vi "robotFollowsHuman.vi"() -> ()   [LabVIEW 2012]
doc: "Simple demonstration of the Kinesthesia toolkit which allows user to conect the Kinect sensor to LabVIEW"
uses:
  <vilib>/LabVIEW Interface for Arduino/Type Defs/Connection Type.ctl
  E:/Kinect/Neobotix/CSInterface/RosBridgeDotNet.dll
  RosBridgeDotNet.dll
  <vilib>/University of Leeds/Kinesthesia Toolkit for Microsoft Kinect/_Polymorphic Close/Close-Skeleton and Video.vi
  <vilib>/University of Leeds/Kinesthesia Toolkit for Microsoft Kinect/_Polymorphic Configure/Event-Skeleton and Video.vi
  <vilib>/University of Leeds/Kinesthesia Toolkit for Microsoft Kinect/_Polymorphic Read/Read-Skeleton and Video.vi
  <vilib>/LabVIEW Interface for Arduino/LabVIEW Interface for Arduino.lvlib
panel:
  in  "Sebesseg":dbl(slide)=1.5254237288135593 scale=1.0..3.0
  in  "Mozog":bool=TRUE
  out "error out":errorcluster
  in  "r":bool
  in  "g":bool
  in  "b":bool
  out "Táv":dbl(slide) scale=0.0..1.4
  out "Szög":dbl(knob)
  out "XY Graph":cluster{"X":dbl[], "Y":dbl[]}[](graph)
  out "y":dbl
  out "x":dbl
  out "Connected":bool
  out "pingelhet":bool
  out "Error Out":errorcluster
  out "Jobb":dbl(slide) scale=-4.0..4.0
  out "Bal":dbl(slide) scale=-4.0..4.0 scale format="%0#1_1g"
  out "2D Picture":picture
  out "3D Skeleton":refnum<vi>(3d-picture)
  in  "stop":bool
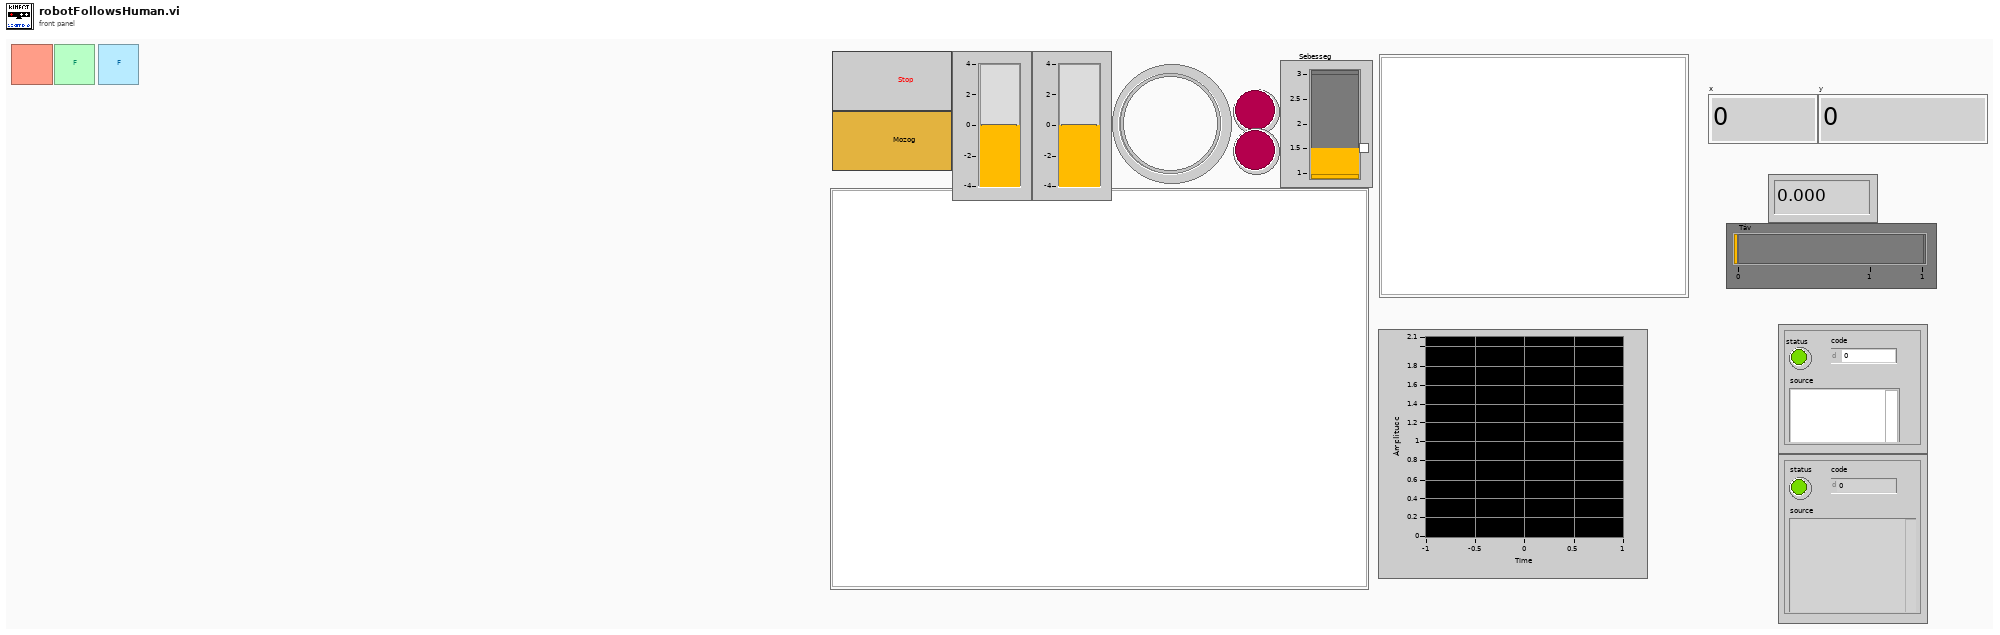
[diagram p1: front panel]
types:
  T1 = typedef "LabVIEW Interface for Arduino.lvlib/Connection Type.ctl" = enum8{"USB / Serial", "XBEE", "BlueSmirf (Bluetooth)"}
  T2 = cluster{cluster{"reference out":refnum<k24>, "KinectSensors":refnum<k24>}, "get_Item":refnum<k24>}
  T3 = cluster{"reference out":refnum<k24>, "KinectSensors":refnum<k24>, "SkeletonStream":refnum<k24>, "ColorStream":refnum<k24>, refnum<k24>[], "get_Item":refnum<k24>}
  T4 = cluster{"Scene":refnum<vi>, "Joints":refnum<vi>[], "Bones":refnum<vi>[]}
  T5 = typedef "LabVIEW Interface for Arduino.lvlib/Arduino Resource.ctl" = cluster{"VISA resource":refnum<visa-resource-name>, "Board Type":T6, "Connection Type":enum8{"USB / Serial"}, "Bytes Per Packet (15)":u8}
  T6 = typedef "LabVIEW Interface for Arduino.lvlib/Board Type.ctl" = enum16{"Uno", "Dimuelanove w/Atmega 328", "Mega 2560"}
  T7 = enum16{"hip centre", "spine", "shoulder centre", "head", "shoulder left", "elbow left", "wrist left", "hand left", "shoulder right", "elbow right", "wrist right", "hand right", "hip left", "knee left", "ankle left", "foot left", "hip right", "knee right", "ankle right", "foot right"}
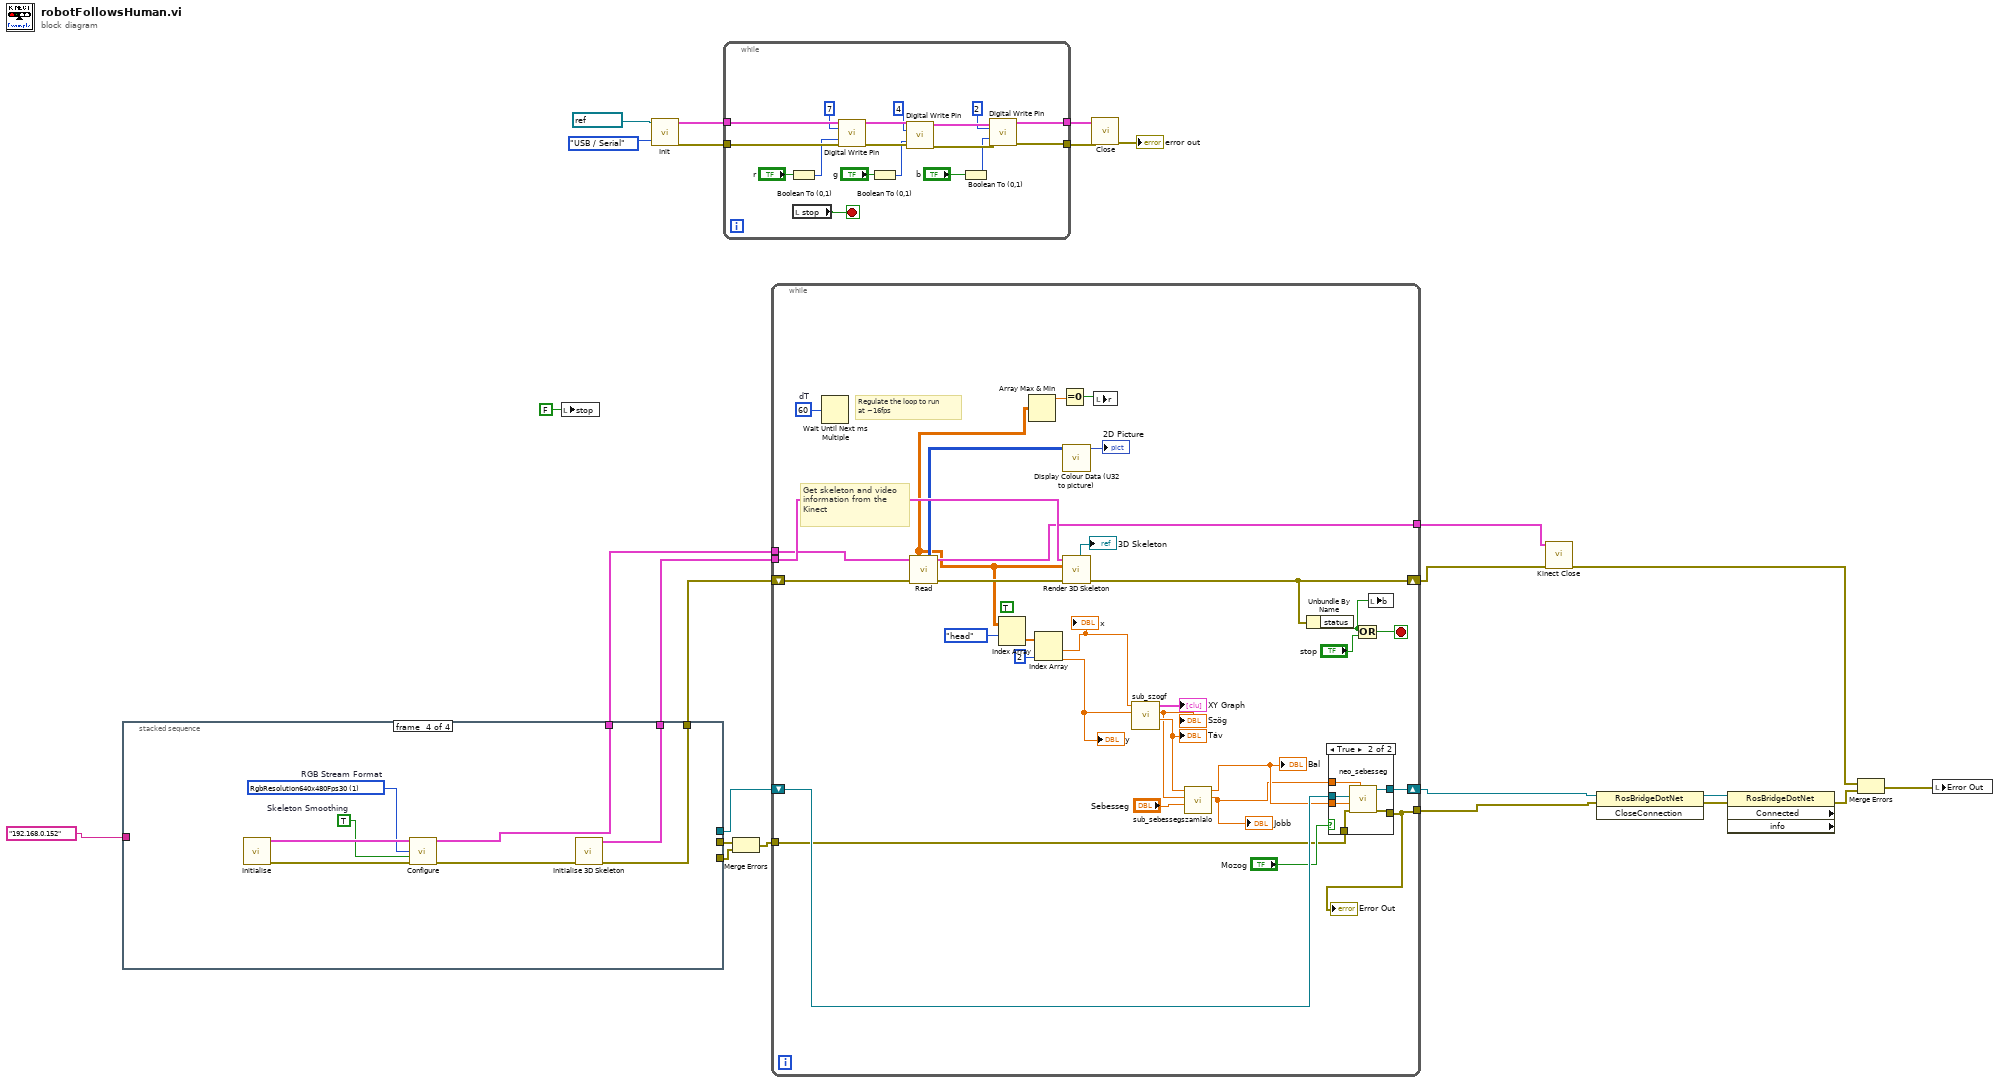
[diagram p0: block diagram]
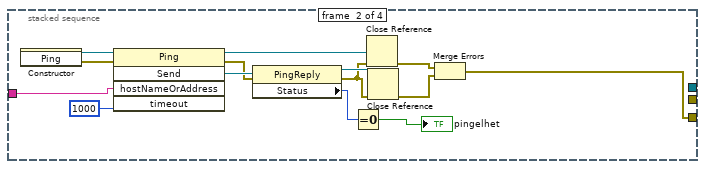
[diagram p3: hidden frame]
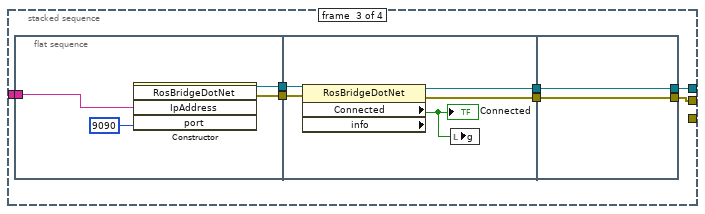
[diagram p4: hidden frame]
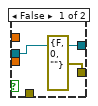
[diagram p5: hidden frame]
diagram:
  n1 = stacked-sequence {
    tunnel: "192.168.0.152" ("IpAddress") -> [_ w33 w42 _]
    tunnel: [_ _ w41 _] -> w21
    tunnel: [_ _ w40 _] -> w9
    tunnel: [_ w26 _ _] -> w7
    tunnel: [_ _ _ w60] -> w6
    tunnel: [_ _ _ w59] -> w5
    tunnel: [_ _ _ w58] -> w4
    frame #0 {
    }
    frame #1 {
      n2 = constructor class="Ping"() -> (reference out=w38:refnum<k24>, error out=w30:errorcluster)  [unwired: 3 in, 1 out]
      n3 = invoke class="Ping" method="Send"(reference=w38, error in=w30, "hostNameOrAddress"=w33, "timeout"=1000) -> (reference out=w36:refnum<k24>, error out=w31:errorcluster, "Send"=w39:refnum<k24>)  [unwired: 1 in, 2 out]
      n4 = property class="PingReply"(reference=w39, error in=w31) -> (reference out=w37:refnum<k24>, error out=w29:errorcluster, "Status"=w34:i32)
      n5 = Equal To 0?(x=w34) -> (x = 0?=→"pingelhet":bool)
      n6 = Close Reference(reference=w36, error in (no error)=w29) -> (error out=w28:errorcluster)
      n7 = Close Reference(reference=w37, error in (no error)=w29) -> (error out=w27:errorcluster)
      n8 = Merge Errors(w28, w27) -> (w26:errorcluster)
    }
    frame #2 {
      n9 = flat-sequence {
        tunnel: [w49] -> w46
        tunnel: [w48] -> w45
        tunnel: w42 -> [w47]
        tunnel: w46 -> [w55]
        tunnel: w45 -> [w54]
        tunnel: [w53] -> w44
        tunnel: [w52] -> w43
        tunnel: w44 -> [w56]
        tunnel: w43 -> [w57]
        tunnel: [w57] -> w40
        tunnel: [w56] -> w41
        frame #0 {
          n10 = constructor class="RosBridgeDotNet"("IpAddress"=w47, "port"=9090) -> (reference out=w49:refnum<k24>, error out=w48:errorcluster)  [unwired: 3 in, 3 out]
        }
        frame #1 {
          n11 = property class="RosBridgeDotNet" props=["Connected", "info"](reference=w55, error in=w54) -> (reference out=w53:refnum<k24>, error out=w52:errorcluster, "Connected"=w51:bool)  [unwired: 1 out]
          "Connected" <- w51
          n12 = local write "g"(w51) -> ()
        }
        frame #2 {
        }
      }
    }
    frame #3 {
      w62 = 1 items=["Undefined", "RgbResolution640x480Fps30", "RgbResolution1280x960Fps12", "YuvResolution640x480Fps15", "RawYuvResolution640x480Fps15"]  # RGB Stream Format
      w63 = TRUE  # Skeleton Smoothing
      n13 = call <vilib>:"Initialise.vi"() -> ("Kinect References out"=w65:T2, "error out"=w64:errorcluster)  [unwired: 14 in]
      n14 = call-poly <vilib>:"Configure.vi"("Kinect References in"=w65, "RGB Stream Format"=w62, "Skeleton Smoothing"=w63, "error in"=w64) -> ("Kinect References out"=w59:T3, "error out"=w61:errorcluster)  [unwired: 10 in]
      n15 = call <vilib>:"Initialise 3D Skeleton.vi"("error in (no error)"=w61) -> ("error out"=w58:errorcluster, "Scene & Skeleton Refs"=w60:T4)  [unwired: 9 in]
    }
  }
  n16 = local write "stop"(FALSE ("stop")) -> ()
  n17 = call <vilib>:"Init.vi"("VISA resource"=refnum<visa-resource-name> "COM3" ("visares"), "Connection Type (USB/Serial)"=Connection_Type."USB / Serial") -> ("Arduino Resource"=w14:T5, "error out"=w13:errorcluster)  [unwired: 16 in]
  n18 = while {
    tunnel: w14 -> [w83]
    tunnel: [w75] -> w11
    tunnel: w13 -> [w82]
    tunnel: [w76] -> w10
    stop <- w66 stop-if-true
    n19 = Boolean To (0,1)(Boolean="r") -> (0, 1=w71:i16)
    n20 = local read "stop"() -> (w66:bool)
    n21 = call <vilib>:"Digital Write Pin.vi"("Arduino Resource"=w83, "Digital I/O Pin (0)"=u8 7, "Value (0)"=w71, "error in"=w82) -> ("Arduino Resource"=w80:T5, "error out"=w79:errorcluster)  [unwired: 10 in]
    n22 = Boolean To (0,1)(Boolean="g") -> (0, 1=w68:i16)
    n23 = call <vilib>:"Digital Write Pin.vi"("Arduino Resource"=w80, "Digital I/O Pin (0)"=u8 4, "Value (0)"=w68, "error in"=w79) -> ("Arduino Resource"=w78:T5, "error out"=w77:errorcluster)  [unwired: 10 in]
    n24 = Boolean To (0,1)(Boolean="b") -> (0, 1=w67:i16)
    n25 = call <vilib>:"Digital Write Pin.vi"("Arduino Resource"=w78, "Digital I/O Pin (0)"=u8 2, "Value (0)"=w67, "error in"=w77) -> ("Arduino Resource"=w75:T5, "error out"=w76:errorcluster)  [unwired: 10 in]
  }
  n26 = Merge Errors(w9, w7) -> (w8:errorcluster)
  n27 = while {
    tunnel: [w106] -> w24
    tunnel: w6 -> [w115]
    tunnel: w5 -> [w107]
    shift-right: [w108] -> w25
    shift-left: w4 -> [w105]
    shift-right: [w100] -> w20
    shift-left: w21 -> [w101]
    tunnel: [w99] -> w19
    tunnel: w8 -> [w85]
    stop <- w109 stop-if-true
    (unwired) TRUE ("Custom Coordinates Instead of Joint 2")
    w113 = u32 60  # dT
    # "Get skeleton and video\ninformation from the Kinect"
    # "Regulate the loop to run\nat ~16fps"
    n28 = Wait Until Next ms Multiple(millisecond multiple=w113) -> ()  [unwired: 1 out]
    n29 = call-poly <vilib>:"Read.vi"("Kinect References in"=w107, "error in (no error)"=w105) -> ("Primary Skeleton Array"=w92:dbl[][], "Colour output array (U24, RGB)"=w93:u32[][], "Kinect References out"=w106:T3, "error out"=w111:errorcluster)  [unwired: 9 in, 1 out]
    n30 = Index Array(array=w92, index (row)=T7."head" ("Joint 1")) -> (element=w103:dbl[])  [unwired: 1 in]
    n31 = Array Max & Min(array=w92) -> (max value=w91:dbl)  [unwired: 3 out]
    n32 = Index Array(array=w103, index #2=2 ("index")) -> (element #1=w98:dbl, element #2=w97:dbl)  [unwired: 1 in]
    "x" <- w98
    "y" <- w97
    n33 = Equal To 0?(x=w91) -> (x = 0?=w90:bool)
    n34 = call <vilib>:"Display Colour Data (U32 to picture).vi"("Colour output array (U24, RGB)"=w93) -> ("new picture"=→"2D Picture":picture)  [unwired: 10 in]
    n35 = call <vilib>:"Render 3D Skeleton.vi"("error in (no error)"=w111, "Array of Joint Positions"=w92, "Scene & Skeleton Refs In"=w115) -> ("error out"=w108:errorcluster, "Scene Out"=→"3D Skeleton":refnum<vi>)  [unwired: 5 in, 2 out]
    n36 = local write "r"(w90) -> ()
    n37 = call "sub_szogf.vi"("y"=w97, "x"=w98) -> ("Táv"=w95:dbl, "SzögNulllpont"=w94:dbl, "XY Graph"=→"XY Graph":cluster{"X":dbl[], "Y":dbl[]}[])  [unwired: 7 in]
    "Szög" <- w94
    "Táv" <- w95
    n38 = call "sub_sebessegszamlalo.vi"("Sebesseg"="Sebesseg", "Szög"=w94, "Táv"=w95) -> ("Jobb"=w87:dbl, "Bal"=w88:dbl)  [unwired: 7 in]
    "Bal" <- w88
    "Jobb" <- w87
    n39 = Unbundle By Name(w108) -> ("status"=w89:bool)
    n40 = case shown="True" "Mozog" {
      tunnel: w101 -> [w117 w123]
      tunnel: [w117 w122] -> w100
      tunnel: [errorcluster {"status"=FALSE, "code"=0, "source"=""} ("error out") w121] -> w99
      tunnel: w88 -> [_ w120]
      tunnel: w87 -> [_ w119]
      tunnel: w85 -> [_ w118]
      frame False {
      }
      frame True {
        n41 = call "neo_sebesseg.vi"("Jobb"=w119, "error in (no error)"=w118, "Bal"=w120, "new reference in"=w123) -> ("error out"=w121:errorcluster, ".NET Refnum out"=w122:refnum<k24>)  [unwired: 5 in, 1 out]
      }
    }
    "Error Out" <- w99
    n42 = Or(x=w89, y="stop") -> (x .or. y?=w109:bool)
    n43 = local write "b"(w89) -> ()
  }
  n44 = call <vilib>:"Close.vi"("Arduino Resource"=w11, "error in"=w10) -> ("error out"=→"error out":errorcluster)  [unwired: 13 in]
  n45 = call-poly <vilib>:"Kinect Close.vi"("Kinect References in"=w24, "error in"=w25) -> ("error out"=w2:errorcluster)  [unwired: 13 in]
  n46 = invoke class="RosBridgeDotNet" method="CloseConnection"(reference=w20, error in=w19) -> (reference out=w17:refnum<k24>, error out=w18:errorcluster)  [unwired: 1 in, 1 out]
  n47 = property class="RosBridgeDotNet" props=["Connected", "info"](reference=w17, error in=w18) -> (error out=w3:errorcluster)  [unwired: 3 out]
  n48 = Merge Errors(w2, w3) -> (w1:errorcluster)
  n49 = local write "Error Out"(w1) -> ()
